vi "Process First Collision.vi"(11 "Game Board in":refnum<class "Game Board.lvclass">) -> (3 "Game Board out":refnum<class "Game Board.lvclass">, 4 "empty collision?":bool)   [LabVIEW 2024, in "Game Board.lvclass"]
doc: "MIT Licence\nCopyright (c) 2024 David Grollier"
uses:
  Game Board.lvclass
  Game Board.lvclass/Game Board.ctl
  Game Board Component/Game Board Component.lvclass/Game Board Component.ctl
  Collision/Collision.lvclass
  Game Board Component/Game Board Component.lvclass
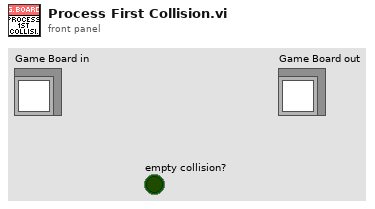
[diagram p1: front panel]
types:
  T1 = map{string, refnum<class "Game Board Component.lvclass">}
  T2 = cluster{"Dichotomie factor":dbl, "Collision":refnum<class "Collision.lvclass">}[]
  T3 = cluster{"Dichotomie factor":dbl, "Collision":refnum<class "Collision.lvclass">}
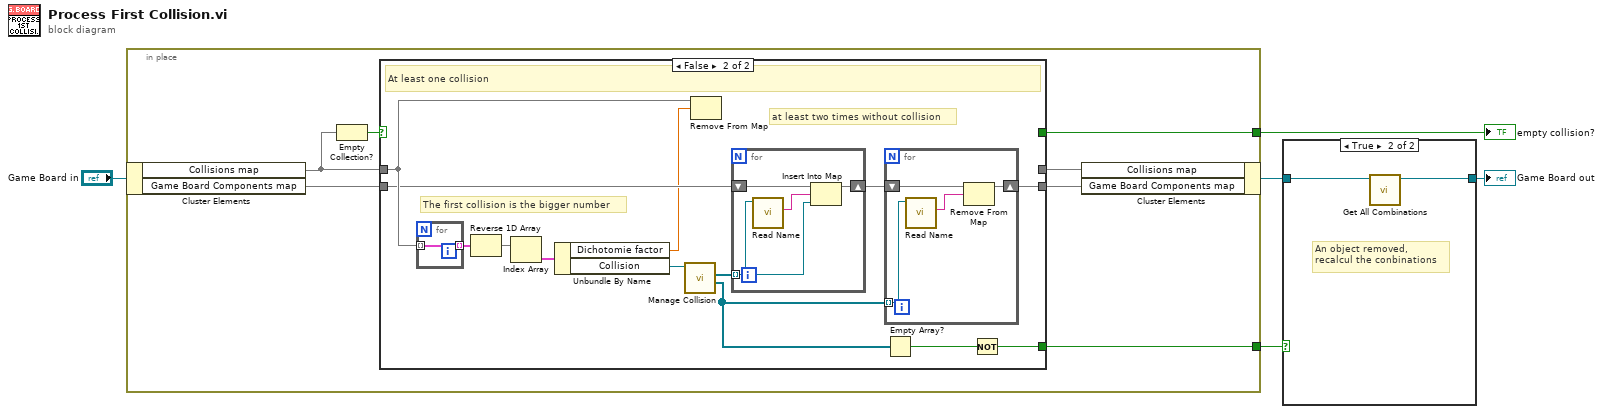
[diagram p0: block diagram]
diagram:
  n1 = in-place {
    in-place-border: [w9] -> w5
    in-place-border: [w6] -> w3
    n2 = in-place-cluster #1("Game Board in") -> ("Collisions map"=w7:map{dbl, refnum<class "Collision.lvclass">}, "Game Board Components map"=w12:T1)
    n3 = Empty Collection?(1:w7) -> (0:w8:bool)
    n4 = case shown="False" w8 {
      selector: w8 -> [w13 _]
      tunnel: w12 -> [w14 w26]
      tunnel: [w14 w19] -> w11
      tunnel: [w15 _] -> w10
      tunnel: w7 -> [w15 w28]
      tunnel: [w13 _] -> w9
      tunnel: [_ w16] -> w6
      frame True {
      }
      frame False {
        # "The first collision is the bigger number"
        # "at least two times without collision"
        # "At least one collision"
        n5 = for {
          tunnel: w28 -> [w33] mode=indexing
          tunnel: [w33] -> w25 mode=indexing
        }
        n6 = Reverse 1D Array(array=w25) -> (reversed array=w24:T2)
        n7 = Index Array(array=w24) -> (element=w23:T3)  [unwired: 1 in]
        n8 = Unbundle By Name(w23) -> ("Dichotomie factor"=w21:dbl, "Collision"=w22:refnum<class "Collision.lvclass">)
        n9 = call-dynamic "Manage Collision.vi"("Collision in"=w22) -> ("Remove GB Components out"=w18:refnum<class "Game Board Component.lvclass">[], "Insert GB Components out"=w27:refnum<class "Game Board Component.lvclass">[])  [unwired: 9 in]
        n10 = Remove From Map(10:w21, 11:w28) -> ()  [unwired: 3 out]
        n11 = for {
          shift-right: [w31] -> w20
          shift-left: w26 -> [w32]
          tunnel: w27 -> [w29] mode=indexing
          n12 = call "Read Name.vi"("Game Board Component in"=w29) -> ("Name"=w30:string)  [unwired: 10 in]
          n13 = Insert Into Map(map in=w32, key=w30, value=w29) -> (map out=w31:T1)  [unwired: 2 out]
        }
        n14 = for {
          shift-right: [w37] -> w19
          shift-left: w20 -> [w34]
          tunnel: w18 -> [w36] mode=indexing
          n15 = call "Read Name.vi"("Game Board Component in"=w36) -> ("Name"=w35:string)  [unwired: 10 in]
          n16 = Remove From Map(10:w35, 11:w34) -> (3:w37:T1)  [unwired: 2 out]
        }
        n17 = Empty Array?(array=w18) -> (empty?=w17:bool)
        n18 = Not(x=w17) -> (.not. x?=w16:bool)
      }
    }
    n19 = in-place-cluster #1("Collisions map"=w10, "Game Board Components map"=w11) -> (w2:refnum<class "Game Board.lvclass">)
  }
  "empty collision?" <- w5
  n20 = case shown="True" w3 {
    tunnel: w2 -> [w38 w40]
    tunnel: [w38 w39] -> w1
    frame False {
    }
    frame True {
      # "An object removed,\nrecalcul the conbinations"
      n21 = call "Get All Combinations.vi"("Game Board in"=w40) -> ("Game Board out"=w39:refnum<class "Game Board.lvclass">)  [unwired: 10 in]
    }
  }
  "Game Board out" <- w1
